vi "Get RIOs and Channels List.vi"(8 "error in (no error)":errorcluster, 9 "rio names":string[](array[string]), 10 "ip list property name":string, 11 "Item Ref in":T2 format="%.0x") -> (0 "error out":errorcluster, 2 "rios and channels":T1(array[cluster]), 3 "Item Ref out":T2 format="%.0x")   [LabVIEW 2015, in "Engine Simulation Toolkit System Explorer.lvlib"]
uses:
  Engine Simulation Toolkit System Explorer.lvlib
  <vilib>/NI Veristand/Custom Device API/Custom Device Item Ref.ctl
  <vilib>/NI Veristand/Custom Device Tools/Custom Device Utility Library/Search Direction.ctl
  Shared/Constants and GUIDs.vi
  <vilib>/NI Veristand/Custom Device Tools/Custom Device Utility Library/NI VeriStand - Search for Item by GUID.vi
  <vilib>/NI Veristand/Custom Device API/Get Item Property (String Array).vi
  <vilib>/NI Veristand/Custom Device Tools/Custom Device Utility Library/Custom Device Utility Library.lvlib
  Shared/Engine Simulation Toolkit Shared.lvlib
  <vilib>/NI Veristand/Custom Device API/Custom Device API.lvlib
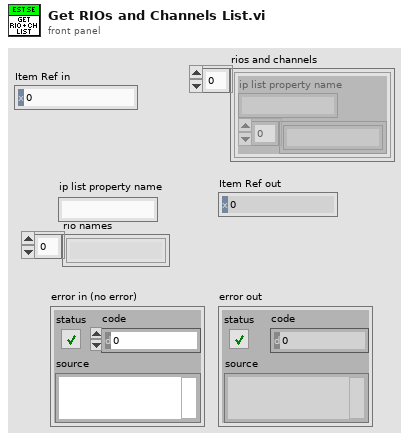
[diagram p1: front panel]
types:
  T1 = cluster{"ip list property name":string, string[]}[]
  T2 = typedef "Custom Device API.lvlib/Custom Device Item Ref.ctl" = u64
  T3 = typedef "Custom Device Utility Library.lvlib/Search Direction.ctl" = enum16{"Down", "Up"}
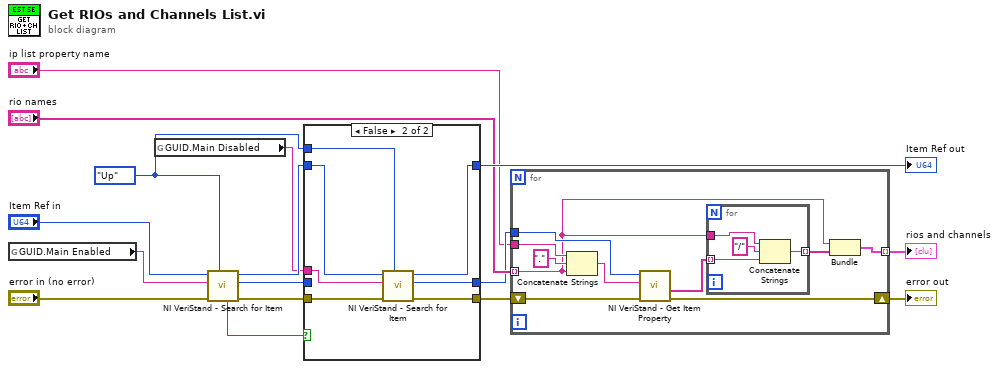
[diagram p0: block diagram]
diagram:
  w8 = Search_Direction."Up" ("Direction (Down)")
  n1 = global read "Constants and GUIDs.vi" "GUID.Main Enabled"() -> (w14:string)
  n2 = global read "Constants and GUIDs.vi" "GUID.Main Disabled"() -> (w9:string)
  n3 = call-poly <vilib>:"NI VeriStand - Search for Item.vi"("Direction (Down)"=w8, "error in"="error in (no error)", "Item GUID"=w14, "Section Ref in"="Item Ref in") -> ("error out"=w12:errorcluster, "Item Ref"=w10:T2, "Section Ref out"=w11:T2, "Found"=w13:bool)  [unwired: 4 in]
  n4 = case shown="False" w13 {
    tunnel: w12 -> [w19 w26]
    tunnel: w11 -> [w17 w25]
    tunnel: w10 -> [w18 _]
    tunnel: w9 -> [_ w24]
    tunnel: w8 -> [_ w23]
    tunnel: [w18 w22] -> w5
    tunnel: [w17 w21] -> w7
    tunnel: [w19 w20] -> w4
    frame True {
    }
    frame False {
      n5 = call-poly <vilib>:"NI VeriStand - Search for Item.vi"("Direction (Down)"=w23, "error in"=w26, "Item GUID"=w24, "Section Ref in"=w25) -> ("error out"=w20:errorcluster, "Item Ref"=w22:T2, "Section Ref out"=w21:T2)  [unwired: 4 in, 1 out]
    }
  }
  "Item Ref out" <- w7
  n6 = for {
    tunnel: "rio names" -> [w27] mode=indexing
    tunnel: w5 -> [w36]
    shift-right: [w34] -> w3
    shift-left: w4 -> [w35]
    tunnel: "ip list property name" -> [w28]
    tunnel: [w29] -> w1 mode=indexing
    n7 = Concatenate Strings(w28, "." ("string"), w27) -> (w32:string)
    n8 = call-poly <vilib>:"NI VeriStand - Get Item Property.vi"("error in (no error)"=w35, "Property Name"=w32, "Item Ref in"=w36) -> ("error out"=w34:errorcluster, "Value"=w31:string[])  [unwired: 5 in, 2 out]
    n9 = for {
      tunnel: w27 -> [w39]
      tunnel: w31 -> [w38] mode=indexing
      tunnel: [w37] -> w30 mode=indexing
      n10 = Concatenate Strings(w39, "/" ("string"), w38) -> (w37:string)
    }
    n11 = Bundle("String"=w27, w30) -> (w29:cluster{"String":string, string[]})  [unwired: 1 in]
  }
  "error out" <- w3
  "rios and channels" <- w1
